vi "速度及航向.vi"(11 "速度及航向输入":string) -> (2 "航向（度）":sgl, 3 "速度（节）":dbl)   [LabVIEW 2018]
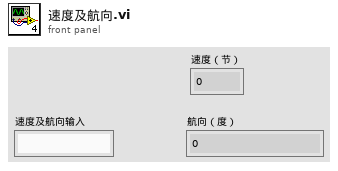
[diagram p1: front panel]
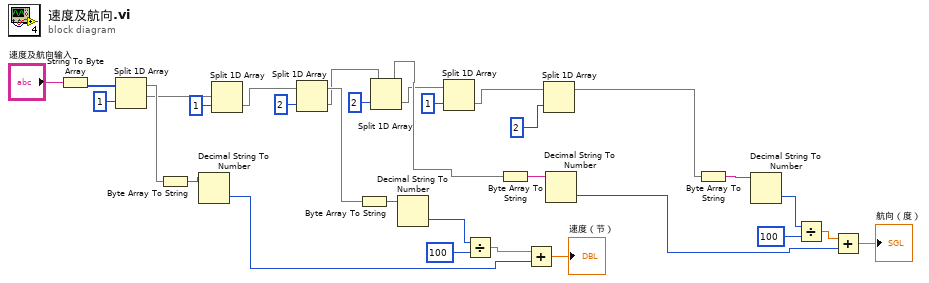
[diagram p0: block diagram]
diagram:
  n1 = String To Byte Array(string="速度及航向输入") -> (unsigned byte array=w9:u8[])
  n2 = Split 1D Array(array=w9, index=1 ("索引")) -> (first subarray=w16:u8[], second subarray=w11:u8[])
  n3 = Byte Array To String(unsigned byte array=w16) -> (string=w15:string)
  n4 = Decimal String To Number(string=w15) -> (number=w25:i32)  [unwired: 2 in, 1 out]
  n5 = Split 1D Array(array=w11, index=1 ("索引")) -> (second subarray=w12:u8[])  [unwired: 1 out]
  n6 = Split 1D Array(array=w12, index=2 ("索引")) -> (first subarray=w20:u8[], second subarray=w13:u8[])
  n7 = Byte Array To String(unsigned byte array=w20) -> (string=w18:string)
  n8 = Split 1D Array(array=w13, index=2 ("索引")) -> (first subarray=w27:u8[], second subarray=w14:u8[])
  n9 = Decimal String To Number(string=w18) -> (number=w22:i32)  [unwired: 2 in, 1 out]
  n10 = Split 1D Array(array=w14, index=1 ("索引")) -> (second subarray=w30:u8[])  [unwired: 1 out]
  n11 = Divide(x=w22, y=100) -> (x/y=w24:dbl)
  n12 = Byte Array To String(unsigned byte array=w27) -> (string=w19:string)
  n13 = Add(x=w24, y=w25) -> (x+y=→"速度（节）":dbl)
  n14 = Split 1D Array(array=w30, index=2 ("索引")) -> (first subarray=w31:u8[])  [unwired: 1 out]
  n15 = Decimal String To Number(string=w19) -> (number=w26:i32)  [unwired: 2 in, 1 out]
  n16 = Byte Array To String(unsigned byte array=w31) -> (string=w17:string)
  n17 = Decimal String To Number(string=w17) -> (number=w21:i32)  [unwired: 2 in, 1 out]
  n18 = Divide(x=w21, y=100) -> (x/y=w23:dbl)
  n19 = Add(x=w23, y=w26) -> (x+y=→"航向（度）":dbl)
